vi "Validation Class.vi"() -> ()   [LabVIEW 2020, in "Library Instrument & Equipement.lvlib" / "Library FireBase.lvlib" / "Firebase AssembledProducts P1817.lvclass"]
uses:
  Firebase AssembledProducts P1817.lvclass
  C:/Users/ngarcin/OneDrive - Altyor/Standard TB/Class/Firebase/Source/Firebase Driver/Firebase Driver.lvclass
  Firebase AssembledProducts P1817.lvclass/Firebase AssembledProducts P1817.ctl
panel:
  out "Get_Data_With_Condition":T1(array[cluster])
  out "Get_Sub_Collection":T2(array[cluster])
  out "tableau ajouté":T3(array[cluster])
  out "Get_Data":T3(array[cluster])
  out "sortie d'erreur":errorcluster
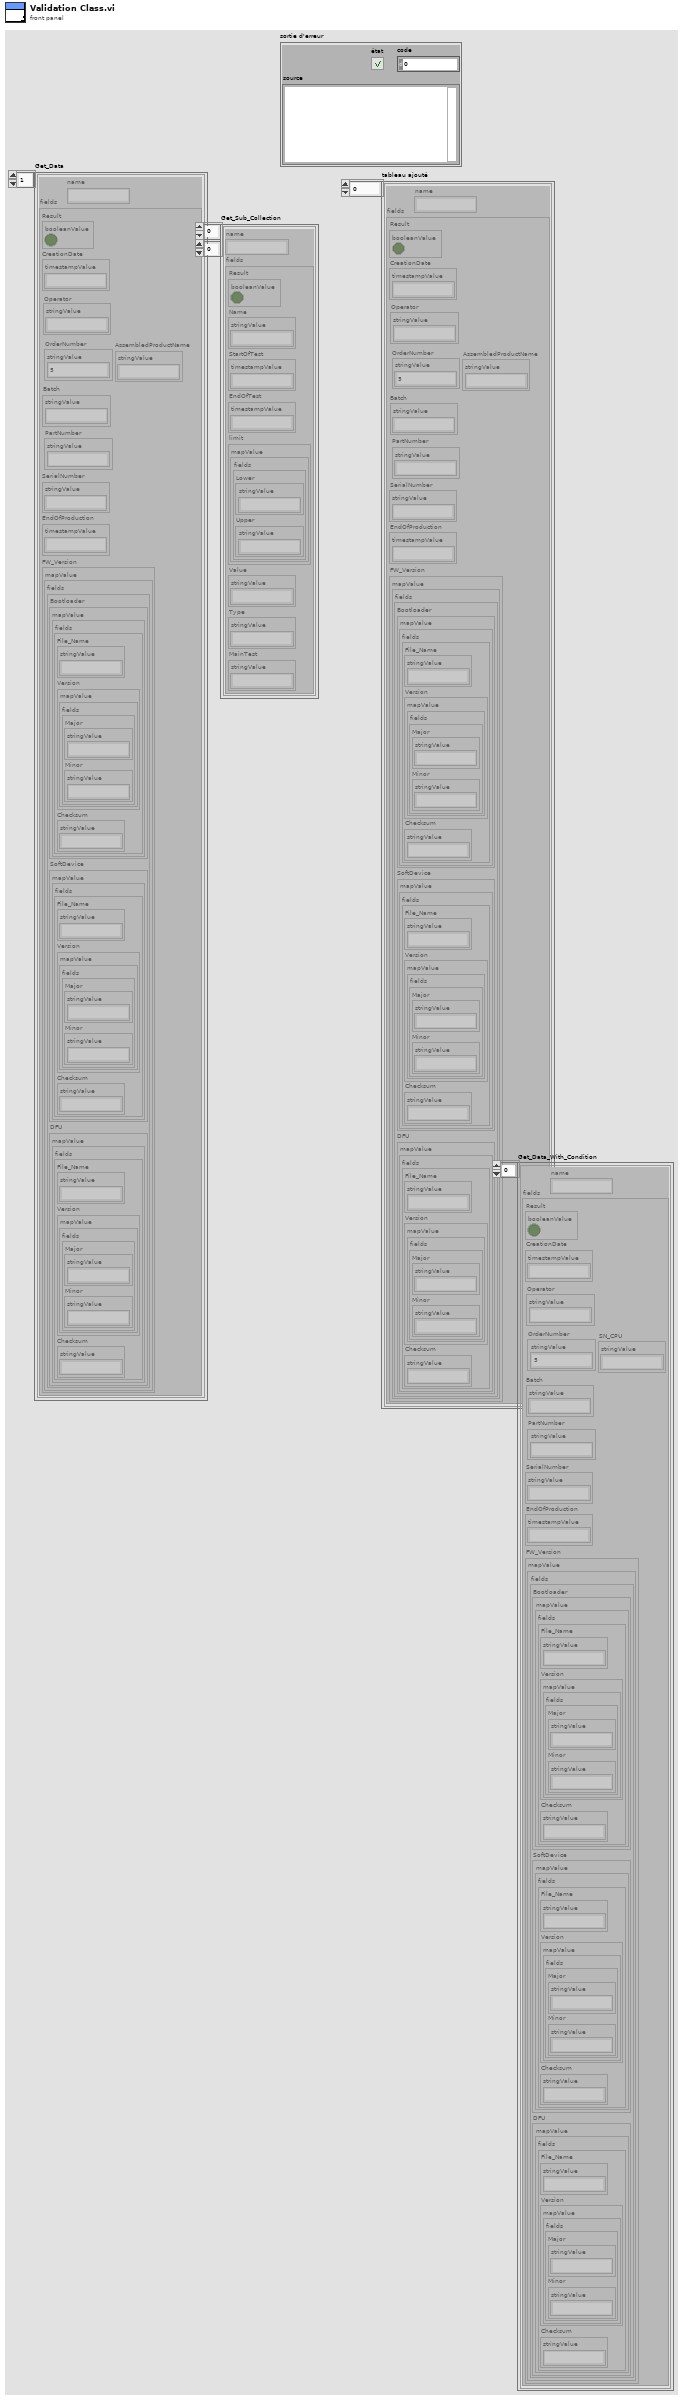
[diagram p1: front panel]
types:
  T1 = cluster{"name":string, "fields":cluster{"Result":cluster{"booleanValue":bool}, "CreationDate":cluster{"timestampValue":string}, "Batch":cluster{"stringValue":string}, "SerialNumber":cluster{"stringValue":string}, "EndOfProduction":cluster{"timestampValue":string}, "FW_Version":cluster{"mapValue":cluster{"fields":cluster{"Bootloader":cluster{"mapValue":cluster{"fields":cluster{"File_Name":cluster{"stringValue":string}, "Version":cluster{"mapValue":cluster{"fields":cluster{"Major":cluster{"stringValue":string}, "Minor":cluster{"stringValue":string}}}}, "Checksum":cluster{"stringValue":string}}}}, "SoftDevice":cluster{"mapValue":cluster{"fields":cluster{"File_Name":cluster{"stringValue":string}, "Version":cluster{"mapValue":cluster{"fields":cluster{"Major":cluster{"stringValue":string}, "Minor":cluster{"stringValue":string}}}}, "Checksum":cluster{"stringValue":string}}}}, "DFU":cluster{"mapValue":cluster{"fields":cluster{"File_Name":cluster{"stringValue":string}, "Version":cluster{"mapValue":cluster{"fields":cluster{"Major":cluster{"stringValue":string}, "Minor":cluster{"stringValue":string}}}}, "Checksum":cluster{"stringValue":string}}}}}}}, "PartNumber":cluster{"stringValue":string}, "OrderNumber":cluster{"stringValue":string}, "Operator":cluster{"stringValue":string}, "SN_CPU":cluster{"stringValue":string}}}[]
  T2 = cluster{"name":string, "fields":cluster{"Result":cluster{"booleanValue":bool}, "Name":cluster{"stringValue":string}, "StartOfTest":cluster{"timestampValue":string}, "EndOfTest":cluster{"timestampValue":string}, "limit":cluster{"mapValue":cluster{"fields":cluster{"Lower":cluster{"stringValue":string}, "Upper":cluster{"stringValue":string}}}}, "Value":cluster{"stringValue":string}, "Type":cluster{"stringValue":string}, "MainTest":cluster{"stringValue":string}}}[][]
  T3 = cluster{"name":string, "fields":cluster{"Result":cluster{"booleanValue":bool}, "CreationDate":cluster{"timestampValue":string}, "Batch":cluster{"stringValue":string}, "SerialNumber":cluster{"stringValue":string}, "EndOfProduction":cluster{"timestampValue":string}, "FW_Version":cluster{"mapValue":cluster{"fields":cluster{"Bootloader":cluster{"mapValue":cluster{"fields":cluster{"File_Name":cluster{"stringValue":string}, "Version":cluster{"mapValue":cluster{"fields":cluster{"Major":cluster{"stringValue":string}, "Minor":cluster{"stringValue":string}}}}, "Checksum":cluster{"stringValue":string}}}}, "SoftDevice":cluster{"mapValue":cluster{"fields":cluster{"File_Name":cluster{"stringValue":string}, "Version":cluster{"mapValue":cluster{"fields":cluster{"Major":cluster{"stringValue":string}, "Minor":cluster{"stringValue":string}}}}, "Checksum":cluster{"stringValue":string}}}}, "DFU":cluster{"mapValue":cluster{"fields":cluster{"File_Name":cluster{"stringValue":string}, "Version":cluster{"mapValue":cluster{"fields":cluster{"Major":cluster{"stringValue":string}, "Minor":cluster{"stringValue":string}}}}, "Checksum":cluster{"stringValue":string}}}}}}}, "PartNumber":cluster{"stringValue":string}, "OrderNumber":cluster{"stringValue":string}, "Operator":cluster{"stringValue":string}, "AssembledProductName":cluster{"stringValue":string}}}[]
  T4 = cluster{"Result":cluster{"booleanValue":bool}, "CreationDate":cluster{"timestampValue":string}, "Batch":cluster{"stringValue":string}, "SerialNumber":cluster{"stringValue":string}, "EndOfProduction":cluster{"timestampValue":string}, "FW_Version":cluster{"mapValue":cluster{"fields":cluster{"Bootloader":cluster{"mapValue":cluster{"fields":cluster{"File_Name":cluster{"stringValue":string}, "Version":cluster{"mapValue":cluster{"fields":cluster{"Major":cluster{"stringValue":string}, "Minor":cluster{"stringValue":string}}}}, "Checksum":cluster{"stringValue":string}}}}, "SoftDevice":cluster{"mapValue":cluster{"fields":cluster{"File_Name":cluster{"stringValue":string}, "Version":cluster{"mapValue":cluster{"fields":cluster{"Major":cluster{"stringValue":string}, "Minor":cluster{"stringValue":string}}}}, "Checksum":cluster{"stringValue":string}}}}, "DFU":cluster{"mapValue":cluster{"fields":cluster{"File_Name":cluster{"stringValue":string}, "Version":cluster{"mapValue":cluster{"fields":cluster{"Major":cluster{"stringValue":string}, "Minor":cluster{"stringValue":string}}}}, "Checksum":cluster{"stringValue":string}}}}}}}, "PartNumber":cluster{"stringValue":string}, "OrderNumber":cluster{"stringValue":string}, "Operator":cluster{"stringValue":string}, "AssembledProductName":cluster{"stringValue":string}, "Delivery":cluster{"booleanValue":bool}}
  T5 = cluster{"Result":cluster{"booleanValue":bool}, "Name":cluster{"stringValue":string}, "StartOfTest":cluster{"timestampValue":string}, "EndOfTest":cluster{"timestampValue":string}, "limit":cluster{"mapValue":cluster{"fields":cluster{"Lower":cluster{"stringValue":string}, "Upper":cluster{"stringValue":string}}}}, "Value":cluster{"stringValue":string}, "Type":cluster{"stringValue":string}, "MainTest":cluster{"stringValue":string}}
  T6 = cluster{"name":string, "fields":cluster{"Result":cluster{"booleanValue":bool}, "CreationDate":cluster{"timestampValue":string}, "Batch":cluster{"stringValue":string}, "SerialNumber":cluster{"stringValue":string}, "EndOfProduction":cluster{"timestampValue":string}, "FW_Version":cluster{"mapValue":cluster{"fields":cluster{"Bootloader":cluster{"mapValue":cluster{"fields":cluster{"File_Name":cluster{"stringValue":string}, "Version":cluster{"mapValue":cluster{"fields":cluster{"Major":cluster{"stringValue":string}, "Minor":cluster{"stringValue":string}}}}, "Checksum":cluster{"stringValue":string}}}}, "SoftDevice":cluster{"mapValue":cluster{"fields":cluster{"File_Name":cluster{"stringValue":string}, "Version":cluster{"mapValue":cluster{"fields":cluster{"Major":cluster{"stringValue":string}, "Minor":cluster{"stringValue":string}}}}, "Checksum":cluster{"stringValue":string}}}}, "DFU":cluster{"mapValue":cluster{"fields":cluster{"File_Name":cluster{"stringValue":string}, "Version":cluster{"mapValue":cluster{"fields":cluster{"Major":cluster{"stringValue":string}, "Minor":cluster{"stringValue":string}}}}, "Checksum":cluster{"stringValue":string}}}}}}}, "PartNumber":cluster{"stringValue":string}, "OrderNumber":cluster{"stringValue":string}, "Operator":cluster{"stringValue":string}, "AssembledProductName":cluster{"stringValue":string}, "Delivery":cluster{"booleanValue":bool}}}[]
  T7 = cluster{"Result":cluster{"booleanValue":bool}, "CreationDate":cluster{"timestampValue":string}, "Batch":cluster{"stringValue":string}, "SerialNumber":cluster{"stringValue":string}, "EndOfProduction":cluster{"timestampValue":string}, "FW_Version":cluster{"mapValue":cluster{"fields":cluster{"Bootloader":cluster{"mapValue":cluster{"fields":cluster{"File_Name":cluster{"stringValue":string}, "Version":cluster{"mapValue":cluster{"fields":cluster{"Major":cluster{"stringValue":string}, "Minor":cluster{"stringValue":string}}}}, "Checksum":cluster{"stringValue":string}}}}, "SoftDevice":cluster{"mapValue":cluster{"fields":cluster{"File_Name":cluster{"stringValue":string}, "Version":cluster{"mapValue":cluster{"fields":cluster{"Major":cluster{"stringValue":string}, "Minor":cluster{"stringValue":string}}}}, "Checksum":cluster{"stringValue":string}}}}, "DFU":cluster{"mapValue":cluster{"fields":cluster{"File_Name":cluster{"stringValue":string}, "Version":cluster{"mapValue":cluster{"fields":cluster{"Major":cluster{"stringValue":string}, "Minor":cluster{"stringValue":string}}}}, "Checksum":cluster{"stringValue":string}}}}}}}, "PartNumber":cluster{"stringValue":string}, "OrderNumber":cluster{"stringValue":string}, "Operator":cluster{"stringValue":string}, "SN_CPU":cluster{"stringValue":string}}
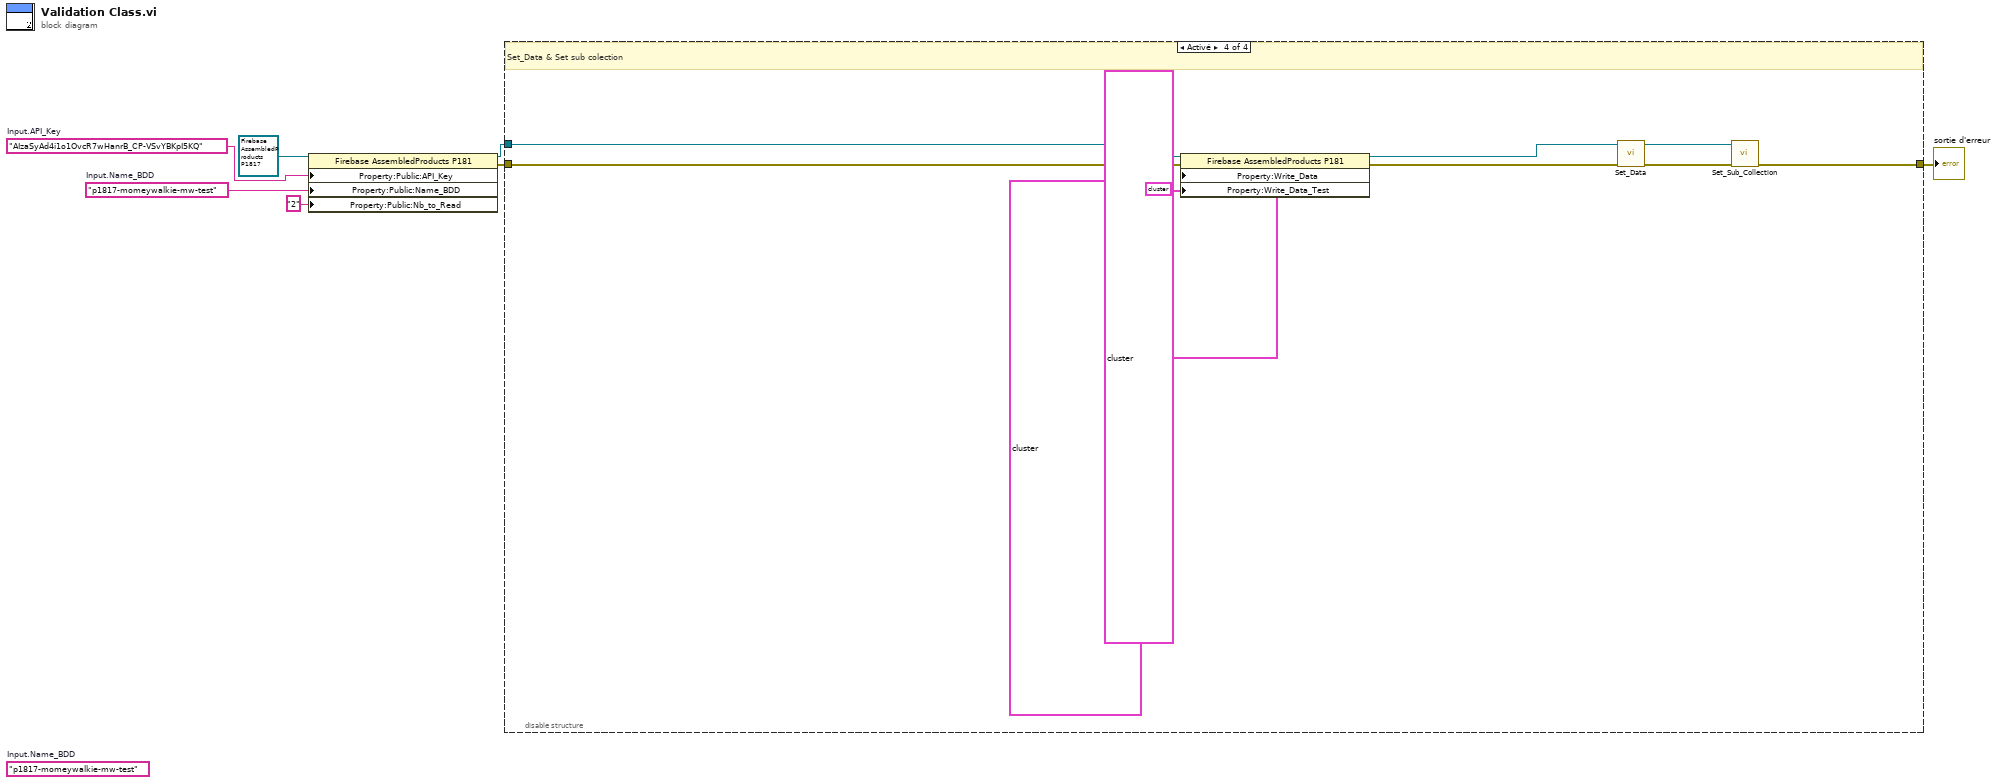
[diagram p0: block diagram]
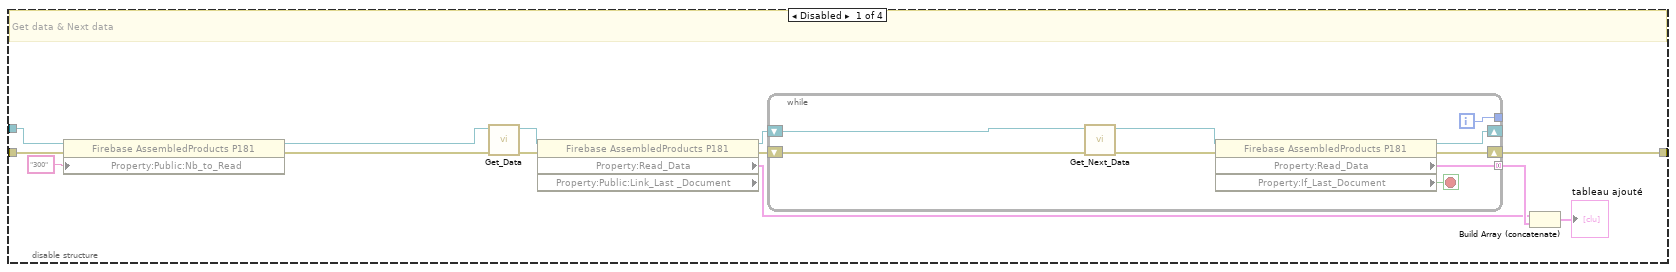
[diagram p2: hidden frame]
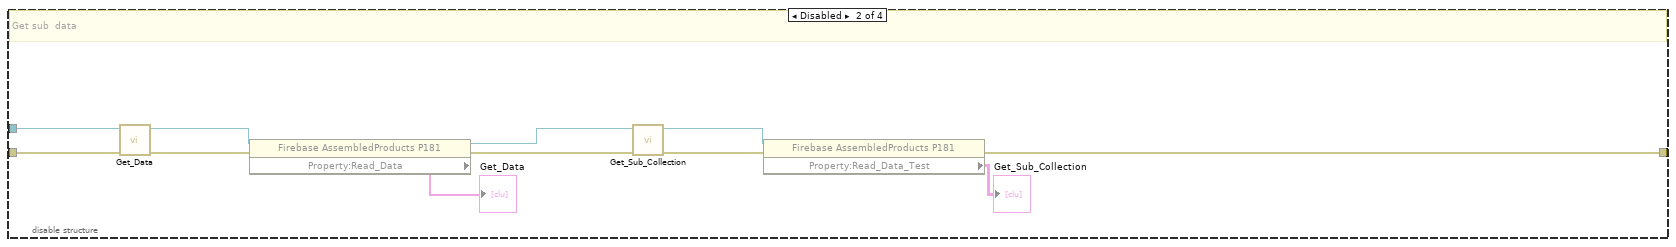
[diagram p3: hidden frame]
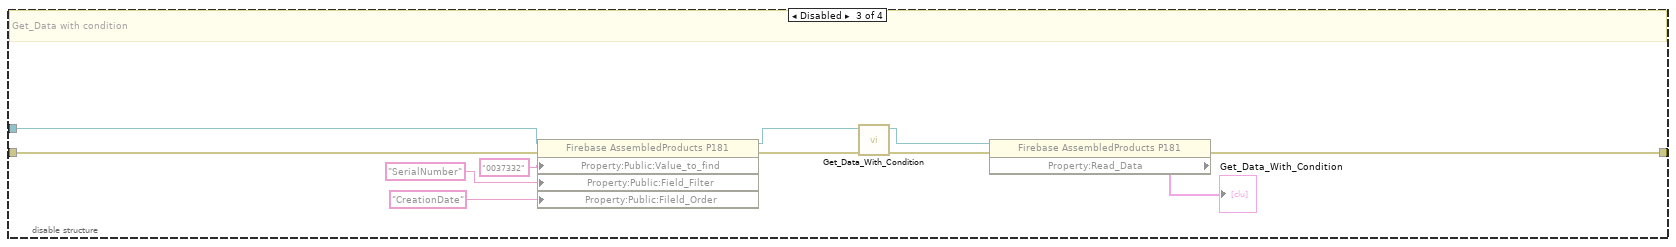
[diagram p4: hidden frame]
diagram:
  w3 = "AIzaSyAd4i1o1OvcR7wHanrB_CP-VSvYBKpI5KQ"  # Input.API_Key
  (unwired) "p1817-momeywalkie-mw-test"  # Input.Name_BDD
  w2 = "p1817-momeywalkie-mw-test"  # Input.Name_BDD
  n1 = property class="Firebase AssembledProducts P181"(reference=refnum<class "Firebase AssembledProducts P1817.lvclass"> refnum ("Build Library FireBase.lvlib:Firebase AssembledProducts.lvclass"), "Property:Public:API_Key"=w3, "Property:Public:Name_BDD"=w2, "Property:Public:Nb_to_Read"="2" ("Nb_to_Read")) -> (reference out=w4:refnum<class "Firebase AssembledProducts P1817.lvclass">, error out=w5:errorcluster)  [unwired: 1 in]
  n2 = disable-structure shown="Activé" {
    disable-tunnel: [w20 w40 w43 w55] -> w6
    disable-tunnel: w5 -> [w10 w34 w41 w54]
    disable-tunnel: w4 -> [w12 w32 w42 w53]
    frame Disabled {
      # "Get data & Next data"
      n3 = property class="Firebase AssembledProducts P181"(reference=w12, error in=w10, "Property:Public:Nb_to_Read"="300" ("Nb_to_Read")) -> (reference out=w11:refnum<class "Firebase AssembledProducts P1817.lvclass">, error out=w9:errorcluster)
      n4 = call-dynamic "Get_Data.vi"("error in (no error)"=w9, "Firebase Benches en entrée"=w11) -> ("error out"=w17:errorcluster, "Firebase Benches en sortie"=w16:refnum<class "Firebase AssembledProducts P1817.lvclass">)  [unwired: 8 in]
      n5 = property class="Firebase AssembledProducts P181" props=["Property:Read_Data", "Property:Public:Link_Last _Document"](reference=w16, error in=w17) -> (reference out=w15:refnum<class "Firebase AssembledProducts P1817.lvclass">, error out=w14:errorcluster, "Property:Read_Data"=w13:T6)  [unwired: 1 out]
      n6 = while {
        shift-right: [w29] -> w20
        shift-left: w14 -> [w22]
        tunnel: [w26] -> w19 mode=concatenating
        shift-right: [w28] -> _
        shift-left: w15 -> [w24]
        tunnel: [w27] -> _
        i -> [w27]
        stop <- w25 stop-if-true
        n7 = call-dynamic "Get_Next_Data.vi"("error in (no error)"=w22, "Firebase Benches en entrée"=w24) -> ("error out"=w21:errorcluster, "Firebase Benches en sortie"=w23:refnum<class "Firebase AssembledProducts P1817.lvclass">)  [unwired: 8 in]
        n8 = property class="Firebase AssembledProducts P181"(reference=w23, error in=w21) -> (reference out=w28:refnum<class "Firebase AssembledProducts P1817.lvclass">, error out=w29:errorcluster, "Property:Read_Data"=w26:T6, "Property:If_Last_Document"=w25:bool)
      }
      n9 = Build Array (concatenate)(w13, w19) -> (→"tableau ajouté":T6)
    }
    frame Disabled {
      # "Get sub  data"
      n10 = call-dynamic "Get_Data.vi"("error in (no error)"=w34, "Firebase Benches en entrée"=w32) -> ("error out"=w33:errorcluster, "Firebase Benches en sortie"=w31:refnum<class "Firebase AssembledProducts P1817.lvclass">)  [unwired: 8 in]
      n11 = property class="Firebase AssembledProducts P181"(reference=w31, error in=w33) -> (reference out=w38:refnum<class "Firebase AssembledProducts P1817.lvclass">, error out=w37:errorcluster, "Property:Read_Data"=→"Get_Data":T6)
      n12 = call-dynamic "Get_Sub_Collection.vi"("error in (no error)"=w37, "Firebase Benches en entrée"=w38) -> ("error out"=w36:errorcluster, "Firebase Benches en sortie"=w35:refnum<class "Firebase AssembledProducts P1817.lvclass">)  [unwired: 8 in]
      n13 = property class="Firebase AssembledProducts P181"(reference=w35, error in=w36) -> (error out=w40:errorcluster, "Property:Read_Data_Test"=→"Get_Sub_Collection":T2)  [unwired: 1 out]
    }
    frame Disabled {
      # "Get_Data with condition"
      n14 = property class="Firebase AssembledProducts P181"(reference=w42, error in=w41, "Property:Public:Value_to_find"="0037332" ("Value_to_find"), "Property:Public:Field_Filter"="SerialNumber" ("Field_Filter"), "Property:Public:Fileld_Order"="CreationDate" ("Fileld_Order")) -> (reference out=w48:refnum<class "Firebase AssembledProducts P1817.lvclass">, error out=w47:errorcluster)
      n15 = call-dynamic "Get_Data_With_Condition.vi"("error in (no error)"=w47, "Firebase Benches en entrée"=w48) -> ("error out"=w44:errorcluster, "Firebase Benches en sortie"=w46:refnum<class "Firebase AssembledProducts P1817.lvclass">)  [unwired: 8 in]
      n16 = property class="Firebase AssembledProducts P181"(reference=w46, error in=w44) -> (error out=w43:errorcluster, "Property:Read_Data"=→"Get_Data_With_Condition":T6)  [unwired: 1 out]
    }
    frame Enabled {
      (unwired) T7 {"Result"={"booleanValue"=TRUE}, "CreationDate"={"timestampValue"="2023-06-13T16:56:05.299Z"}, "Batch"={"stringValue"=""}, "SerialNumber"={"stringValue"="EP26160514"}, "EndOfProduction"={"timestampValue"="2023-06-13T16:56:05.299Z"}, "FW_Version"={"mapValue"={"fields"={"Bootloader"={"mapValue"={"fields"={"File_Name"={"stringValue"=""}, "Version"={"mapValue"={"fields"={"Major"={"stringValue"=""}, "Minor"={"stringValue"=""}}}}, "Checksum"={"stringValue"=""}}}}, "SoftDevice"={"mapValue"={"fields"={"File_Name"={"stringValue"=""}, "Version"={"mapValue"={"fields"={"Major"={"stringValue"=""}, "Minor"={"stringValue"=""}}}}, "Checksum"={"stringValue"=""}}}}, "DFU"={"mapValue"={"fields"={"File_Name"={"stringValue"=""}, "Version"={"mapValue"={"fields"={"Major"={"stringValue"=""}, "Minor"={"stringValue"=""}}}}, "Checksum"={"stringValue"=""}}}}}}}, "PartNumber"={"stringValue"="048454542"}, "OrderNumber"={"stringValue"=""}, "Operator"={"stringValue"="Nothing"}, "SN_CPU"={"stringValue"=""}} ("fields")
      # "Set_Data & Set sub colection"
      n17 = property class="Firebase AssembledProducts P181"(reference=w53, error in=w54, "Property:Write_Data"=T4 {"Result"={"booleanValue"=FALSE}, "CreationDate"={"timestampValue"=""}, "Batch"={"stringValue"=""}, "SerialNumber"={"stringValue"=""}, "EndOfProduction"={"timestampValue"=""}, "FW_Version"={"mapValue"={"fields"={"Bootloader"={"mapValue"={"fields"={"File_Name"={"stringValue"=""}, "Version"={"mapValue"={"fields"={"Major"={"stringValue"=""}, "Minor"={"stringValue"=""}}}}, "Checksum"={"stringValue"=""}}}}, "SoftDevice"={"mapValue"={"fields"={"File_Name"={"stringValue"=""}, "Version"={"mapValue"={"fields"={"Major"={"stringValue"=""}, "Minor"={"stringValue"=""}}}}, "Checksum"={"stringValue"=""}}}}, "DFU"={"mapValue"={"fields"={"File_Name"={"stringValue"=""}, "Version"={"mapValue"={"fields"={"Major"={"stringValue"=""}, "Minor"={"stringValue"=""}}}}, "Checksum"={"stringValue"=""}}}}}}}, "PartNumber"={"stringValue"=""}, "OrderNumber"={"stringValue"="5"}, "Operator"={"stringValue"=""}, "AssembledProductName"={"stringValue"=""}, "Delivery"={"booleanValue"=FALSE}} ("Write_Data"), "Property:Write_Data_Test"=T5 {"Result"={"booleanValue"=TRUE}, "Name"={"stringValue"="Position"}, "StartOfTest"={"timestampValue"="2023-06-13T16:56:05.299Z"}, "EndOfTest"={"timestampValue"="2023-06-13T16:56:05.299Z"}, "limit"={"mapValue"={"fields"={"Lower"={"stringValue"=""}, "Upper"={"stringValue"=""}}}}, "Value"={"stringValue"="B10"}, "Type"={"stringValue"="String  "}, "MainTest"={"stringValue"=""}} ("fields")) -> (reference out=w59:refnum<class "Firebase AssembledProducts P1817.lvclass">, error out=w58:errorcluster)
      n18 = call-dynamic "Set_Data.vi"("error in (no error)"=w58, "Firebase Benches en entrée"=w59) -> ("error out"=w56:errorcluster, "Firebase Benches en sortie"=w57:refnum<class "Firebase AssembledProducts P1817.lvclass">)  [unwired: 8 in]
      n19 = call-dynamic "Set_Sub_Collection.vi"("error in (no error)"=w56, "Firebase PCBA en entrée"=w57) -> ("error out"=w55:errorcluster)  [unwired: 8 in, 1 out]
    }
  }
  "sortie d'erreur" <- w6
